vi "Actor Core.vi"(8 "error in":errorcluster, 11 "Test-Client in":refnum<class "Test-Client.lvclass">) -> (0 "error out":errorcluster, 3 "Actor out":refnum<class "Actor.lvclass">)   [LabVIEW 2020, in "Test-Client.lvlib" / "Test-Client.lvclass"]
doc: "(<B>Filename</B>: Actor Framework.lvlib:Actor.lvclass:Actor Core.vi)\n\nReceives messages to the actor, reacts to them, and initiates any error handling that may shut the actor down.\n\nDescendant classes may override this VI to append parallel tasks for the actor to complete while it handles messages. Overrides use the Call Parent Class Method node."
uses:
  Test-Client.lvclass
  C:/Program Files (x86)/National Instruments/LabVIEW 2020/vi.lib/ActorFramework/Actor/Actor.lvclass
  <vilib>/ActorFramework/Actor/Actor.lvclass
  Test-Client Messages/Popup Msg/Popup Msg.lvclass
  C:/Users/taylo/Projects/LabVIEW/ActorMailbox/MailboxManager/MailBoxMessage/MailBoxMessage.lvclass
  <vilib>/ActorFramework/Actor/Actor.lvclass/Actor.ctl
  <vilib>/ActorFramework/Message Enqueuer/Message Enqueuer.lvclass/Message Enqueuer.ctl
  Test-Client.lvclass/Test-Client.ctl
  MailboxManager/MailboxManager Messages/SendMessageToMailbox Msg/SendMessageToMailbox Msg.lvclass/SendMessageToMailbox Msg.ctl
  MailboxManager/MailboxManager Messages/UnregisterForMessageSpecificType Msg/UnregisterForMessageSpecificType Msg.lvclass/UnregisterForMessageSpecificType Msg.ctl
  <vilib>/ActorFramework/Message Enqueuer/Init from Existing Queue.vi
  <vilib>/ActorFramework/Message Enqueuer/Enqueue.vi
  MailboxManager/MailboxManager Messages/SendMessageToMailbox Msg/SendMessageToMailbox Msg.lvclass
  C:/Program Files (x86)/National Instruments/LabVIEW 2020/vi.lib/ActorFramework/Message/Message.lvclass
  MailboxManager/MailboxManager Messages/UnregisterForMessageSpecificType Msg/UnregisterForMessageSpecificType Msg.lvclass
  <vilib>/ActorFramework/Message Priority Queue/Priority Enqueue.vi
  <vilib>/ActorFramework/Message Enqueuer/Message Enqueuer.lvclass
  MailboxClient/MailboxClient/MailboxClient.lvclass
  C:/Users/taylo/Projects/LabVIEW/ActorMailbox/Test-Client/Test-Client Messages/Popup Msg/Popup Msg.lvclass
  C:/Users/taylo/Projects/LabVIEW/ActorMailbox/Example/ExternClient/MC-ExternClient/MC-ExternClientInterface/MC-ExternClientInterface.lvclass
  C:/Users/taylo/Projects/LabVIEW/ActorMailbox/MailboxClient/MailboxClient/MailboxClient.lvclass
  C:/Users/taylo/Projects/LabVIEW/ActorMailbox/MailboxClientInterface/MailboxClientInterface.lvclass
  C:/Users/taylo/Projects/LabVIEW/ActorMailbox/Test-Client/Test-Client/Test-Client.lvclass
  C:/Users/taylo/Projects/LabVIEW/ActorMailbox/Test-Client/Test-Client Messages/Popup Msg/Popup.lvclass
  Test-Client Messages/Incriment Msg/Incriment Msg.lvclass
  C:/Users/taylo/Projects/LabVIEW/ActorMailbox/Test-Client/Test-Client Messages/Incriment Msg/Incriment Msg.lvclass
panel:
  in  "Unrege":bool
  out "Counter":dbl
  in  "Send":bool
  in  "String":string
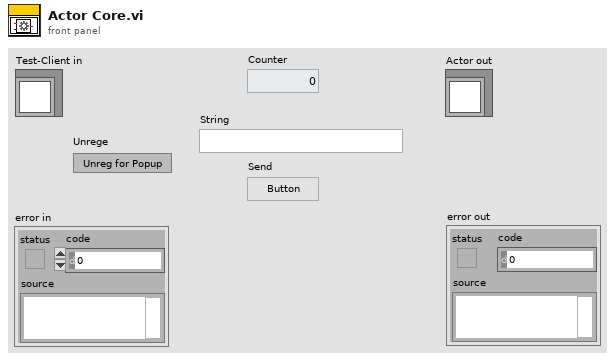
[diagram p1: front panel]
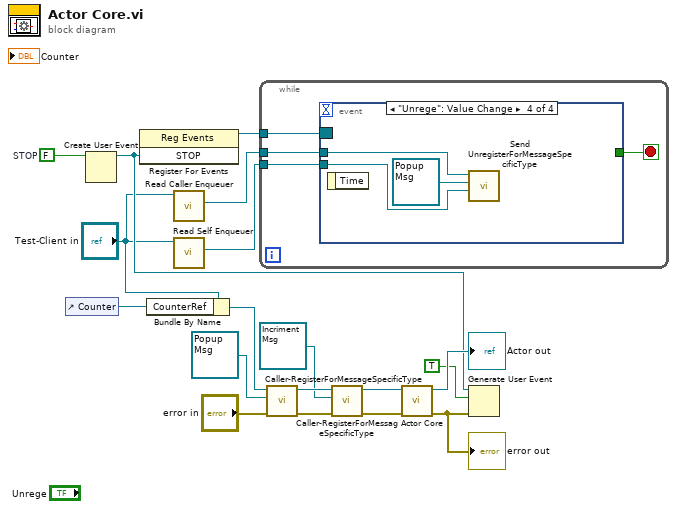
[diagram p0: block diagram]
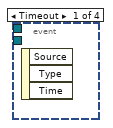
[diagram p2: hidden frame]
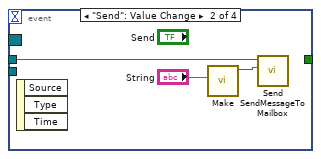
[diagram p3: hidden frame]
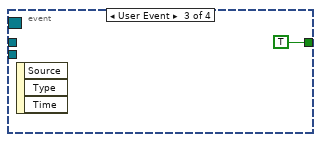
[diagram p4: hidden frame]
diagram:
  w15 = FALSE  # STOP
  n1 = control-ref of="Counter"() -> (w8:refnum<vi>)
  n2 = Create User Event(user event datatype=w15) -> (user event=w12:refnum<user-event>)  [unwired: 1 in, 1 out]
  n3 = register-events(w12) -> (reference out=w14:refnum<event-registration>)  [unwired: 2 in, 1 out]
  n4 = Bundle By Name(cluster="Test-Client in", "CounterRef"=w8) -> (w9:refnum<class "Test-Client.lvclass">)
  n5 = call <vilib>:"Read Caller Enqueuer.vi"("Actor"="Test-Client in") -> ("Caller Enqueuer"=w10:refnum<class "Message Enqueuer.lvclass">)  [unwired: 10 in]
  n6 = call <vilib>:"Read Self Enqueuer.vi"("Actor"="Test-Client in") -> ("Self Enqueuer"=w6:refnum<class "Message Enqueuer.lvclass">)  [unwired: 10 in]
  n7 = while {
    tunnel: w14 -> [w22]
    tunnel: w10 -> [w21]
    tunnel: w6 -> [w19]
    stop <- w20 stop-if-true
    n8 = event shown="[3] \"Unrege\": Value Change" {
      selector: w22 -> [_ _ _ _]
      dyn-events: _ -> [_ _ _ _]
      timeout: _ -> [_ _ _ _]
      tunnel: w21 -> [_ w25 _ w29]
      tunnel: [_ _ TRUE _] -> w20
      tunnel: w19 -> [_ _ _ w27]
      event Timeout {
        n9 = event-data() -> ()  [unwired: 1 in, 3 out]
      }
      event "Send": Value Change {
        n10 = event-data() -> ()  [unwired: 1 in, 3 out]
        n11 = call "Make.vi"("Msg"="String") -> ("Popup Msg out"=w24:refnum<class "Popup Msg.lvclass">)  [unwired: 9 in, 1 out]
        n12 = call "Send SendMessageToMailbox.vi"("MailBoxMessage"=w24, "Message Enqueuer"=w25) -> ()  [unwired: 8 in, 2 out]
      }
      event User Event {
        n13 = event-data() -> ()  [unwired: 1 in, 3 out]
      }
      event "Unrege": Value Change {
        n14 = event-data() -> ()  [unwired: 1 in, 1 out]
        n15 = call "Send UnregisterForMessageSpecificType.vi"("Message Enqueuer 2"=w27, "Message"=refnum<class "Popup Msg.lvclass"> refnum ("Test-Client.lvlib:Popup Msg.lvclass"), "Message Enqueuer"=w29) -> ()  [unwired: 7 in, 2 out]
      }
    }
  }
  n16 = call-dynamic "Caller-RegisterForMessageSpecificType.vi"("error in (no error)"="error in", "MailBoxMessage"=refnum<class "Popup Msg.lvclass"> refnum ("Test-Client.lvlib:Popup Msg.lvclass"), "MailboxClient in"=w9) -> ("error out"=w2:errorcluster, "MailboxClient out"=w5:refnum<class "Test-Client.lvclass">)  [unwired: 7 in]
  n17 = call-dynamic "Caller-RegisterForMessageSpecificType.vi"("error in (no error)"=w2, "MailBoxMessage"=refnum<class "Incriment Msg.lvclass"> refnum ("Test-Client.lvlib:Incriment Msg.lvclass"), "MailboxClient in"=w5) -> ("error out"=w1:errorcluster, "MailboxClient out"=w4:refnum<class "Test-Client.lvclass">)  [unwired: 7 in]
  n18 = call-parent "Actor Core.vi"("error in"=w1, "Actor in"=w4) -> ("error out"=w13:errorcluster, "Actor out"=→"Actor out":refnum<class "Actor.lvclass">)  [unwired: 8 in]
  "error out" <- w13
  n19 = Generate User Event(user event=w12, event data cluster=TRUE ("event data"), error in=w13) -> ()  [unwired: 1 in, 2 out]
